vi "Disabled__LCR.vi"(10 "Control":refnum<vi>) -> (2 "Disabled?":bool)   [LabVIEW 2011, in "BooleanXControl__LCR.xctl"]
doc: "This VI controls the state of the Control, and returns True if it's state is Disabled."
uses:
  BooleanXControl__LCR.xctl
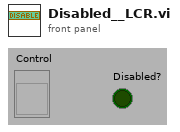
[diagram p1: front panel]
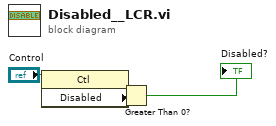
[diagram p0: block diagram]
diagram:
  n1 = property class="Ctl"(reference="Control") -> ("Disabled"=w2:u8)  [unwired: 1 in, 2 out]
  n2 = Greater Than 0?(x=w2) -> (x > 0?=→"Disabled?":bool)
